vi "Create Statement Line.vi"(4 "Time Stamp Format":string="%Y%m%dT%H%M%S%3u", 6 "Delimiter":string=",", 8 "Error In":errorcluster, 11 "Statement":T1) -> (0 "Error Out":errorcluster, 3 "Line":string)   [LabVIEW 2025, in "LOGlib_LV2025.lvlib"]
doc: "Converts a logging statement to a Comma Separated Values (CSV) line."
uses:
  LOGlib_LV2025.lvlib
  Type Definitions/Statement.ctl
  Type Definitions/Tag.ctl
  <vilib>/Utility/error.llb/Trim Whitespace.vi
  <vilib>/dlg_ctls.llb/Space Constant.vi
  <vilib>/Utility/error.llb/Trim Whitespace One-Sided.vi
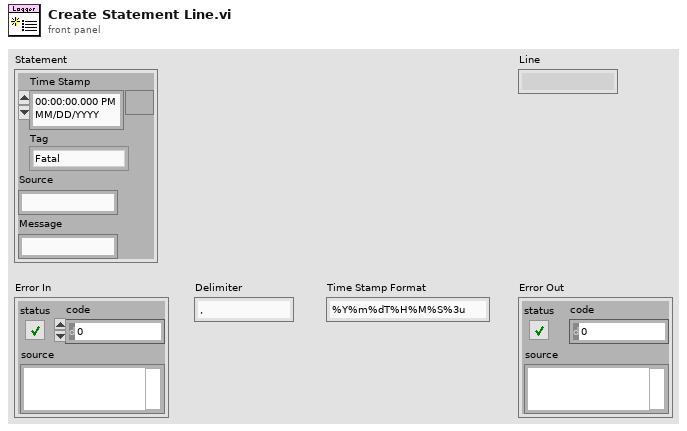
[diagram p1: front panel]
types:
  T1 = typedef "LOGlib_LV2025.lvlib/Statement.ctl" = cluster{"Time Stamp":timestamp, "Tag":T2, "Source":string, "Message":string}
  T2 = typedef "LOGlib_LV2025.lvlib/Tag.ctl" = enum16{"Fatal", "Error", "Warn", "Info", "Debug", "Trace"}
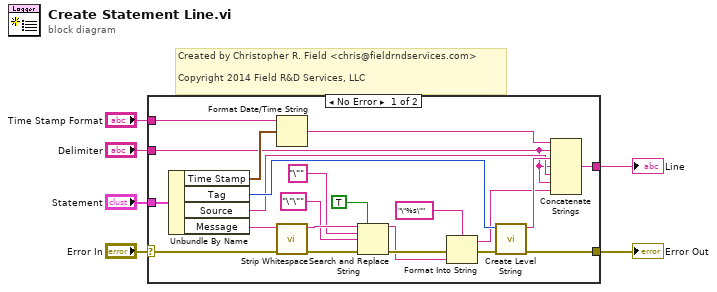
[diagram p0: block diagram]
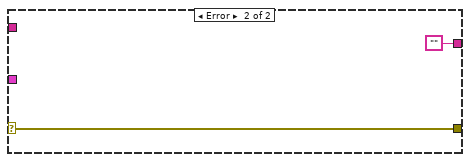
[diagram p2: hidden frame]
diagram:
  # "Created by Christopher R. Field <chris@fieldrndservices.com>\n\nCopyright 2014 Field R&D Services, LLC"
  n1 = case shown="No Error" "Error In" {
    selector: "Error In" -> [w21 w30]
    tunnel: "Statement" -> [w28 _]
    tunnel: [w23 w30] -> w4
    tunnel: [w22 ""] -> w3
    tunnel: "Delimiter" -> [w7 _]
    tunnel: "Time Stamp Format" -> [w9 _]
    frame No Error {
      n2 = Unbundle By Name(w28) -> ("Time Stamp"=w27:timestamp, "Tag"=w26:T2, "Source"=w24:string, "Message"=w20:string)
      n3 = Format Date/Time String(time format string (%c)=w9, seconds (now)=w27) -> (date/time string=w8:string)  [unwired: 1 in]
      n4 = call "Strip Whitespace.vi"("Error In"=w21, "Text"=w20) -> ("Error Out"=w16:errorcluster, "Stripped Text"=w13:string)  [unwired: 8 in]
      n5 = Search and Replace String(replace all?=TRUE ("replace all? (F)"), input string=w13, search string="\"", replace string="\"\"" ("replace string (\"\")"), error in=w16) -> (result string=w14:string, error out=w15:errorcluster)  [unwired: 3 in, 2 out]
      n6 = Format Into String(format string="\"%s\"", error in=w15, w14) -> (resulting string=w17:string, error out=w19:errorcluster)  [unwired: 1 in]
      n7 = call "Create Level String.vi"("Error In"=w19, "Level"=w26) -> ("Error Out"=w23:errorcluster, "String"=w25:string)  [unwired: 8 in]
      n8 = Concatenate Strings(w8, w7, w25, w7, w24, w7, w17) -> (w22:string)
    }
    frame Error {
    }
  }
  "Error Out" <- w4
  "Line" <- w3
